vi "Dwell Time Delay.vi"(8 "error in (no error)":errorcluster, 11 "Reader in":refnum<class "Reader.lvclass">) -> (0 "error out":errorcluster, 3 "Reader out":refnum<class "Reader.lvclass">)   [LabVIEW 2009, in "Reader.lvclass"]
doc: "Delay a predetermined time before taking a data point."
uses:
  Reader.lvclass
  Reader.lvclass/Reader.ctl
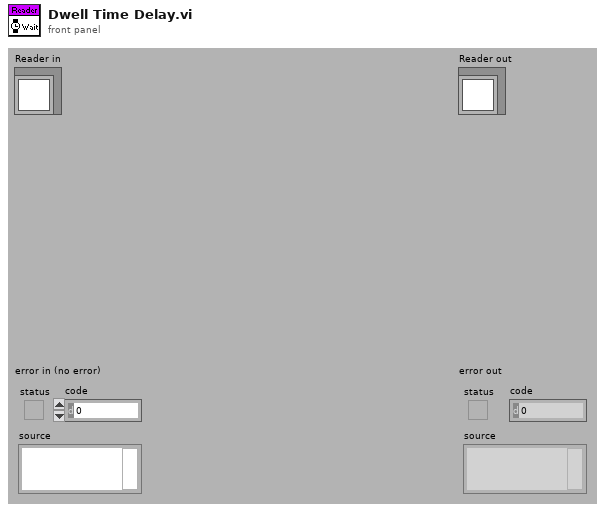
[diagram p1: front panel]
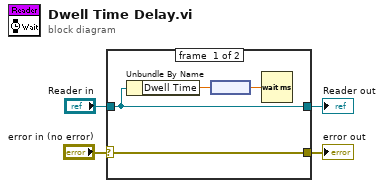
[diagram p0: block diagram]
diagram:
  n1 = case shown="No Error" "error in (no error)" {
    selector: "error in (no error)" -> [w8 w10]
    tunnel: [w8 w10] -> w3
    tunnel: [w6 w9] -> w1
    tunnel: "Reader in" -> [w6 w9]
    frame #0 {
      n2 = Unbundle By Name(w6) -> ("Dwell Time"=w5:dbl[unit])
      n3 = node(w5) -> (w7:dbl)
      n4 = Wait (ms)(milliseconds to wait=w7) -> ()  [unwired: 1 out]
    }
    frame #1 {
    }
  }
  "error out" <- w3
  "Reader out" <- w1
